vi "Close TDMS and Save XML.vi"(8 "error in (no error)":errorcluster, 9 "Logging Queue Cluster":T2, 10 "Exp Params in in":T1 {"period" min=1; "total stacks" min=1; "images per stack" min=1; "total images" min=1; "Z Stack Settings"."Start" min=0.0 max=100.0 step=0.1; "Z Stack Settings"."Step Size" min=0.1 max=100.0 step=0.1; "Z Stack Settings"."Finish" min=0.0 max=100.0 step=0.1; "TSFrames" min=1 step=1; "ZTSdt" min=1 step=1; "ZTSFrames" min=2 step=1; "TSfps" min=1 max=1000 step=1}, 11 "Queue in":refnum<queue>) -> (3 "Review Path":path)   [LabVIEW 2020]
uses:
  _Controls/Logging Queue Cluster.ctl
  _Controls/Tweezertron Ctrl Refs.ctl
  _Controls/Confocal Controls.ctl
  _Controls/iFlex.ctl
  _Controls/PIFOC Position.ctl
  _Controls/Manlight Controls.ctl
  _Controls/Exp Params.ctl
  _Controls/Image Thresholds.ctl
  _Controls/Spots.ctl
  _Controls/Spot Params.ctl
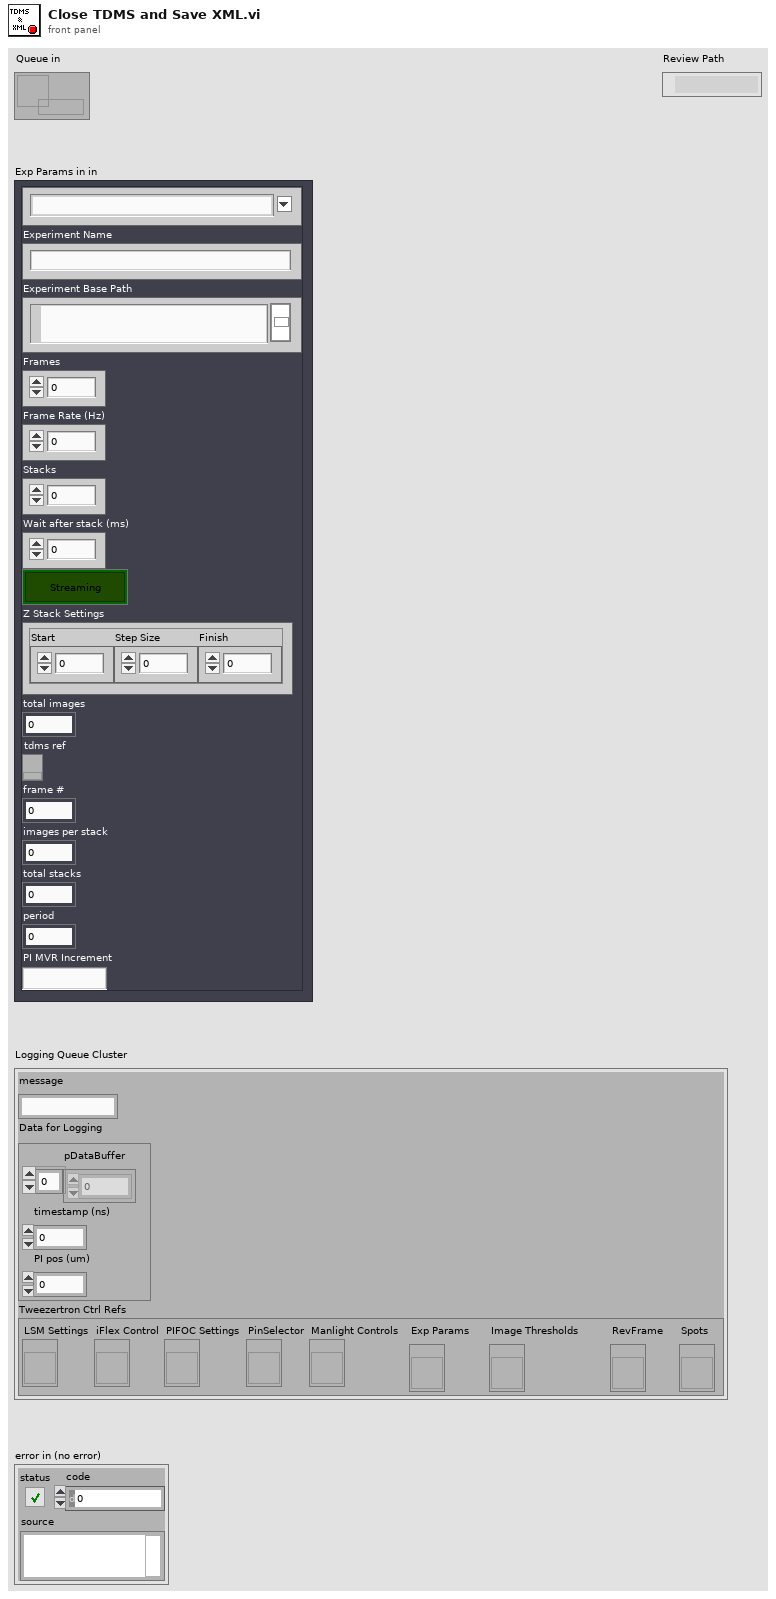
[diagram p1: front panel]
types:
  T1 = typedef "Exp Params.ctl" = cluster{"Experiment Type":string, "Experiment Name":string, "ExpPath":path, "TSFrames":i32, "TSfps":i32, "ZTSFrames":i32, "ZTSdt":i32, "Streaming":bool, "Z Stack Settings":cluster{"Start":dbl, "Step Size":dbl, "Finish":dbl}, "total images":i32, "tdms ref":refnum<k34>, "frame #":i64, "images per stack":i32, "total stacks":i32, "period":i32, "PI MVR Increment":string}
  T2 = typedef "Logging Queue Cluster.ctl" = cluster{"message":string, "Data for Logging":cluster{"pDataBuffer":u16[], "timestamp (ns)":u64, "PI pos (um)":dbl}, "Tweezertron Ctrl Refs":T3}
  T3 = typedef "Tweezertron Ctrl Refs.ctl" = cluster{"LSM Settings":refnum<vi>, "iFlex Control":refnum<vi>, "PIFOC Settings":refnum<vi>, "PinSelector":refnum<vi>, "Manlight Controls":refnum<vi>, "Exp Params":refnum<vi>, "Image Thresholds":refnum<vi>, "RevFrame":refnum<vi>, "Spots":refnum<vi>}
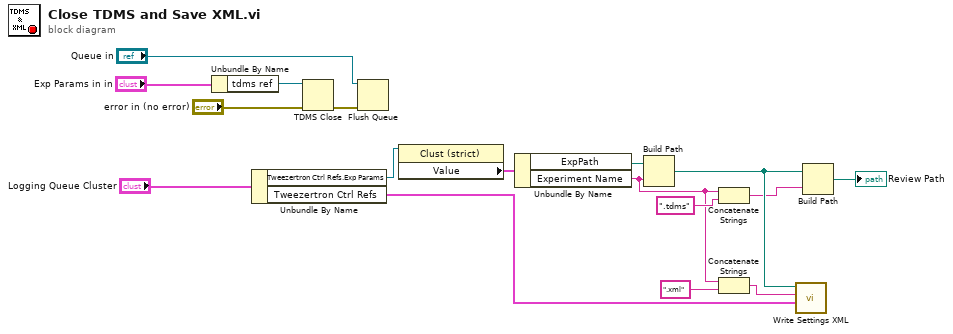
[diagram p0: block diagram]
diagram:
  n1 = Unbundle By Name("Exp Params in in") -> ("tdms ref"=w5:refnum<k34>)
  n2 = Unbundle By Name("Logging Queue Cluster") -> ("Tweezertron Ctrl Refs.Exp Params"=w11:refnum<vi>, "Tweezertron Ctrl Refs"=w14:T3)
  n3 = TDMS Close(8:"error in (no error)", 11:w5) -> (0:w8:errorcluster)  [unwired: 1 out]
  n4 = Flush Queue(queue="Queue in", error in (no error)=w8) -> ()  [unwired: 3 out]
  n5 = property class="Clust (strict)"(reference=w11) -> ("Value"=w12:T1)  [unwired: 1 in, 2 out]
  n6 = Unbundle By Name(w12) -> ("ExpPath"=w15:path, "Experiment Name"=w3:string)
  n7 = Build Path(base path=w15, name or relative path=w3) -> (appended path=w16:path)
  n8 = Concatenate Strings(w3, ".tdms") -> (w10:string)
  n9 = Concatenate Strings(w3, ".xml" ("string")) -> (w1:string)
  n10 = call "Write Settings XML.vi"("Tweezertron Ctrl Refs"=w14, "name or relative path"=w1, "path"=w16) -> ()  [unwired: 8 in, 1 out]
  n11 = Build Path(base path=w16, name or relative path=w10) -> (appended path=→"Review Path":path)
